vi "REPORT_CMPNT_rows_style_pdf.vi"(11 "REPORT_CMPNT_all_info":T1) -> (3 "Row  [ ]":T2)   [LabVIEW 2019]
uses:
  <vilib>/Exaprom PDF/Controls/Table Controls/Table Appearance and Font Row [ ].ctl
  <vilib>/Exaprom PDF/Controls/Table Controls/One Row Appearance.ctl
  <vilib>/Exaprom PDF/Controls/Table Controls/Row from to.ctl
  <vilib>/Exaprom PDF/Controls/Table Controls/Cell, Alignment, LS and Font - hide Vmerge.ctl
  <vilib>/Exaprom PDF/Controls/Table Controls/Cell Type, Alignment and LS.ctl
  <vilib>/Exaprom PDF/Controls/Table Controls/Cell Alignment 20px.ctl
  <vilib>/Exaprom PDF/Controls/Table Controls/Text vertical arrangement.ctl
  <vilib>/Exaprom PDF/Controls/Text Controls/Line spacing.ctl
  <vilib>/Exaprom PDF/Controls/Table Controls/Cell Appearance.ctl
  <vilib>/Exaprom PDF/Controls/Table Controls/Cell Border 20 px.ctl
  <vilib>/Exaprom PDF/Controls/Table Controls/Merge Horizontal.ctl
  <vilib>/Exaprom PDF/Controls/Table Controls/Merge Vertical.ctl
  <vilib>/Exaprom PDF/Controls/Font Controls/Font complete cluster.ctl
  <vilib>/Exaprom PDF/Controls/Font Controls/Font size.ctl
  <vilib>/Exaprom PDF/Controls/Font Controls/Font color.ctl
  <vilib>/Exaprom PDF/Controls/Font Controls/Type and encoding.ctl
  <vilib>/Exaprom PDF/Controls/Text Controls/Unicode/Type and run direction.ctl
  typedef/REPORT_CMPNT_all_info.ctl
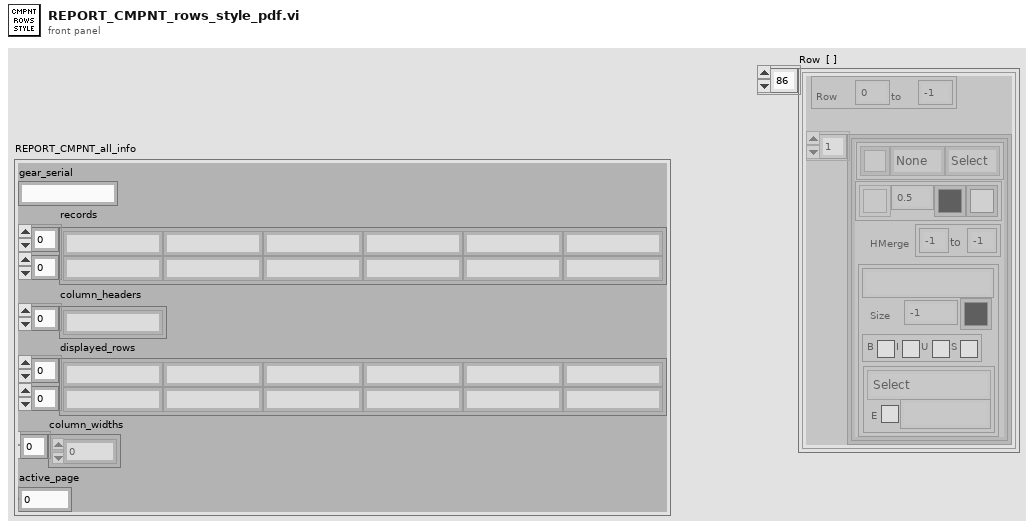
[diagram p1: front panel]
types:
  T1 = typedef "REPORT_CMPNT_all_info.ctl" = cluster{"gear_serial":string, "records":string[][], "column_headers":string[], "displayed_rows":string[][], "column_widths":i16[], "active_page":i32}
  T2 = typedef "Table Appearance and Font Row [ ].ctl" = T3[]
  T3 = typedef "One Row Appearance.ctl" = cluster{"Row":T4, "Cell [ ]":T5[]}
  T4 = typedef "Row from to.ctl" = cluster{"From #":i16, "to #":i16}
  T5 = typedef "Cell, Alignment, LS and Font - hide Vmerge.ctl" = cluster{"Text":T6, "Cell Appearance":T10, "HMerge":T12, "VMerge":T13, "Font":T14}
  T6 = typedef "Cell Type, Alignment and LS.ctl" = cluster{"Cell Alignment":T7, "Text rotation":T8, "Line spacing":T9}
  T7 = typedef "Cell Alignment 20px.ctl" = u16
  T8 = typedef "Text vertical arrangement.ctl" = enum16{"None", "Clockwise", "Counterclockwise"}
  T9 = typedef "Line spacing.ctl" = enum16{"Select", "1.0", "1.5", "2.0"}
  T10 = typedef "Cell Appearance.ctl" = cluster{"Border":T11, "Thickness":sgl, "Color":u32, "BG":u32}
  T11 = typedef "Cell Border 20 px.ctl" = u16
  T12 = typedef "Merge Horizontal.ctl" = cluster{"From":i8, "to":i8}
  T13 = typedef "Merge Vertical.ctl" = cluster{"From":i8, "to":i8}
  T14 = typedef "Font complete cluster.ctl" = cluster{"Name":string, "Size":T15, "Color":T16, "Style":cluster{"Bold":bool, "Italic":bool, "Underline":bool, "Strikeout":bool}, "Type":T17}
  T15 = typedef "Font size.ctl" = sgl
  T16 = typedef "Font color.ctl" = u32
  T17 = typedef "Type and encoding.ctl" = cluster{"Type&direction":T18, "Embedded":bool, "Encoding":string}
  T18 = typedef "Type and run direction.ctl" = enum16{"Select", "ASCII", "UTF-16", "UTF-16 (default)", "UTF-16 (LTR)", "UTF-16 (RTL)"}
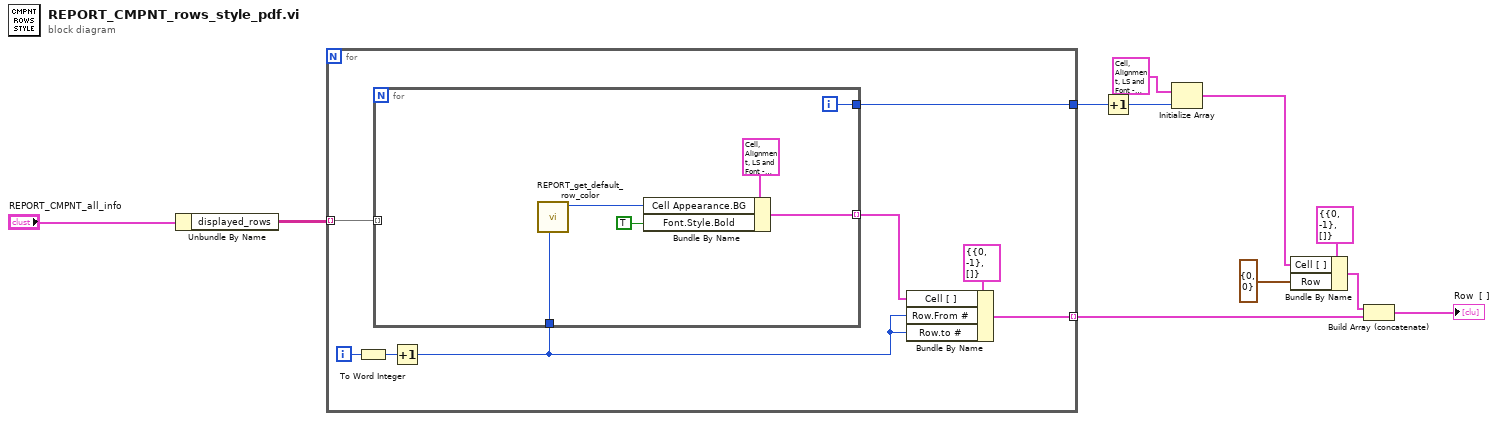
[diagram p0: block diagram]
diagram:
  n1 = Unbundle By Name("REPORT_CMPNT_all_info") -> ("displayed_rows"=w11:string[][])
  n2 = for {
    tunnel: w11 -> [w15] mode=indexing
    tunnel: [w18] -> w9 mode=indexing
    tunnel: [w12] -> w3
    i -> [w17]
    n3 = To Word Integer(number=w17) -> (16bit integer=w16:i16)
    n4 = Increment(x=w16) -> (x+1=w13:i16)
    n5 = for {
      tunnel: w15 -> [_] mode=indexing
      tunnel: [w25] -> w14 mode=indexing
      tunnel: w13 -> [w24]
      tunnel: [w23] -> w12
      i -> [w23]
      n6 = call "REPORT_get_default_row_color.vi"("row"=w24) -> ("color"=w20:u32)  [unwired: 10 in]
      n7 = Bundle By Name(cluster=T5 {"Text"={"Cell Alignment"=0, "Text rotation"=enum."None", "Line spacing"=enum."Select"}, "Cell Appearance"={"Border"=5, "Thickness"=0.5, "Color"=0, "BG"=16448250}, "HMerge"={"From"=-1, "to"=-1}, "VMerge"={"From"=-1, "to"=-1}, "Font"={"Name"="Consolas", "Size"=10.0, "Color"=0, "Style"={"Bold"=FALSE, "Italic"=FALSE, "Underline"=FALSE, "Strikeout"=FALSE}, "Type"={"Type&direction"=enum."ASCII", "Embedded"=FALSE, "Encoding"="CP855"}}} ("Cell, Alignment, LS and Font"), "Cell Appearance.BG"=w20, "Font.Style.Bold"=TRUE ("Active Cell:Cell Font:Bold")) -> (w25:T5)
    }
    n8 = Bundle By Name(cluster=T3 {"Row"={"From #"=0, "to #"=-1}, "Cell [ ]"=[]} ("Row Appearance and Font  [ ]"), "Cell [ ]"=w14, "Row.From #"=w13, "Row.to #"=w13) -> (w18:T3)
  }
  n9 = Increment(x=w3) -> (x+1=w2:i32)
  n10 = Initialize Array(T5 {"Text"={"Cell Alignment"=0, "Text rotation"=enum."None", "Line spacing"=enum."Select"}, "Cell Appearance"={"Border"=5, "Thickness"=1.5, "Color"=16777228, "BG"=16448250}, "HMerge"={"From"=-1, "to"=-1}, "VMerge"={"From"=-1, "to"=-1}, "Font"={"Name"="Consolas", "Size"=10.0, "Color"=16777228, "Style"={"Bold"=TRUE, "Italic"=FALSE, "Underline"=FALSE, "Strikeout"=FALSE}, "Type"={"Type&direction"=enum."ASCII", "Embedded"=FALSE, "Encoding"="CP855"}}} ("Cell, Alignment, LS and Font"), w2) -> (w5:T5[])
  n11 = Bundle By Name(cluster=T3 {"Row"={"From #"=0, "to #"=-1}, "Cell [ ]"=[]} ("Row Appearance and Font  [ ]"), "Cell [ ]"=w5, "Row"=T4 {"From #"=0, "to #"=0}) -> (w7:T3)
  n12 = Build Array (concatenate)(w7, w9) -> (→"Row  [ ]":T3[])
